vi "calibrationElectrometer_acceptCommand_power.vi"(8 "error in (no error)":errorcluster, 11 "command_power_Ctl":T1) -> (0 "error out":errorcluster, 2 "function return":i32, 3 "command_power_Ctl out":T1)   [LabVIEW 2016, in "SALLV_calibrationElectrometer.lvlib"]
doc: "int calibrationElectrometer_shm_acceptCommand_powerLV(calibrationElectrometer_command_powerLV *command_power_Ctl );"
uses:
  SALLV_calibrationElectrometer.lvlib
  DataTypes/command_power.ctl
  SALLV_calibrationElectrometer.so
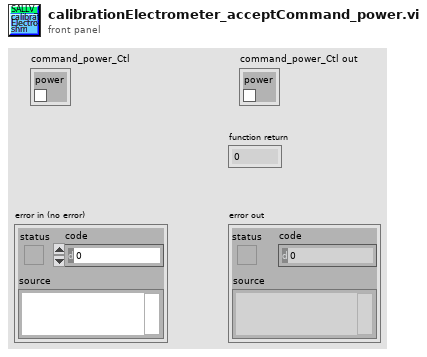
[diagram p1: front panel]
types:
  T1 = typedef "SALLV_calibrationElectrometer.lvlib/command_power.ctl" = cluster{"power":bool}
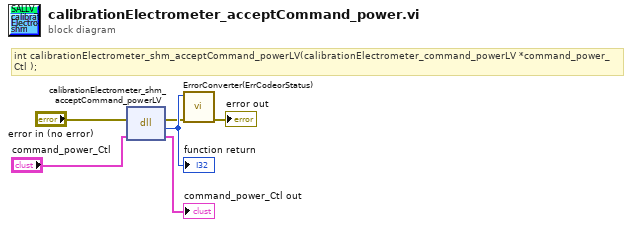
[diagram p0: block diagram]
diagram:
  # "int calibrationElectrometer_shm_acceptCommand_powerLV(calibrationElectrometer_command_powerLV *command_power_Ctl );"
  n1 = dll-call lib="home/andres/Desktop/SAL_calibrationElectrometer/SALLV_calibrationElectrometer.*" fn="calibrationElectrometer_shm_acceptCommand_powerLV"(error in="error in (no error)", "command_power_Ctl"="command_power_Ctl") -> (error out=w2:errorcluster, w6:i32, "command_power_Ctl"=→"command_power_Ctl out":T1)  [unwired: 2 in, 1 out]
  "function return" <- w6
  n2 = call "ErrorConverter(ErrCodeorStatus).vi"("error in (no error)"=w2, "error code"=w6) -> ("error out"=→"error out":errorcluster)  [unwired: 9 in]
